vi "test_scanClocks.vi"() -> ()   [LabVIEW 2016]
uses:
  <vilib>/rvi/DesktopExecutionNode/Execution/niFpgaDEN_Execute.vi
  <vilib>/rvi/DesktopExecutionNode/DesktopExecutionNode.xnode
panel:
  out "moveIndices":cluster{"index":u16, "next":u16}[](array[cluster])
  out "clocks":T1(array[cluster])
  out "fastIndices":cluster{"index":u16, "next":u16}[](array[cluster])
  in  "reset":i32
  in  "moveRates":T2
  in  "scanRates":T3
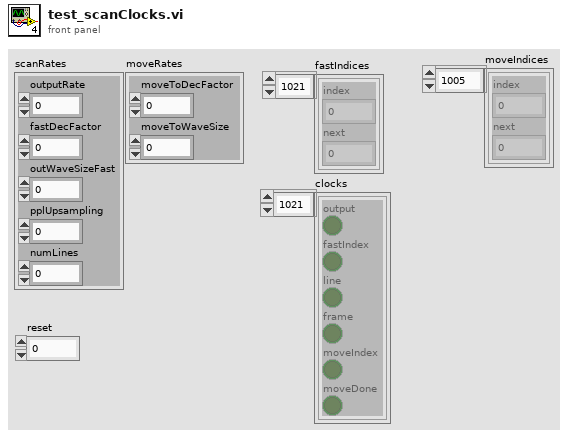
[diagram p1: front panel]
types:
  T1 = cluster{"output":bool, "fastIndex":bool, "line":bool, "frame":bool, "moveIndex":bool, "moveDone":bool}[]
  T2 = cluster{"moveToDecFactor":u16, "moveToWaveSize":u16}
  T3 = cluster{"outputRate":u16, "fastDecFactor":u16, "outWaveSizeFast":u16, "pplUpsampling":u16, "numLines":u16}
  T4 = cluster{"output":bool, "fastIndex":bool, "line":bool, "frame":bool, "moveIndex":bool, "moveDone":bool}
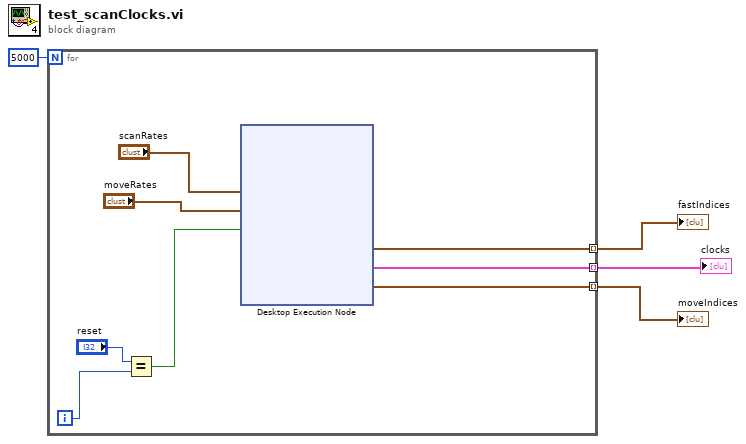
[diagram p0: block diagram]
diagram:
  n1 = for {
    N: 5000 -> [_]
    tunnel: [w7] -> w3 mode=indexing
    tunnel: [w6] -> w2 mode=indexing
    tunnel: [w5] -> w1 mode=indexing
    i -> [w10]
    n2 = Equal?(x="reset", y=w10) -> (x = y?=w8:bool)
    n3 = xnode "Desktop Execution Node"("scanRates"="scanRates", "moveRates"="moveRates", "resetClocks"=w8) -> ("fastIndices"=w7:cluster{"index":u16, "next":u16}, "clocks"=w6:T4, "moveIndices"=w5:cluster{"index":u16, "next":u16})  [unwired: 1 in, 1 out]
  }
  "fastIndices" <- w3
  "clocks" <- w2
  "moveIndices" <- w1
